vi "Enable Disable Controls.vi"(0 "Control Group 1":refnum<vi>[](array[refnum]), 5 "Control Group 2":refnum<vi>[](array[refnum]), 7 "Control Group 3":refnum<vi>[](array[refnum]), 11 "Error In":errorcluster, 12 "Visible / Hidden Control Group 3":bool, 13 "Control Group 2 Mode":T1(ring), 14 "Control Group 1 Mode":T1(ring)) -> (15 "Error Out":errorcluster)   [LabVIEW 2017, in "Waveform-Processing-Custom-Device System Explorer.lvlib"]
doc: "This will receive the reference array from the controls / indicators\nThe first 2 groups will disable/enable/gray/ the control\nThe last group will hide/show the control"
uses:
  Waveform-Processing-Custom-Device System Explorer.lvlib
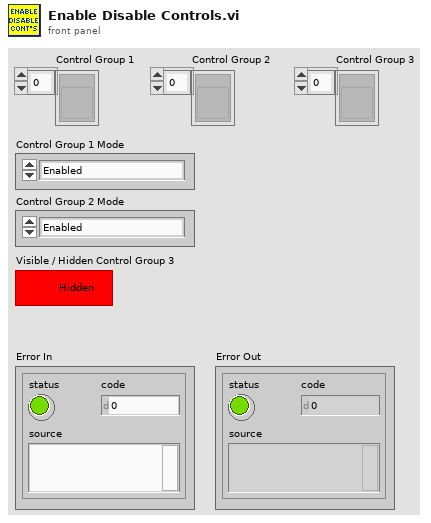
[diagram p1: front panel]
types:
  T1 = enum8{"Enabled", "Disabled", "Disabled and Grayed Out"}
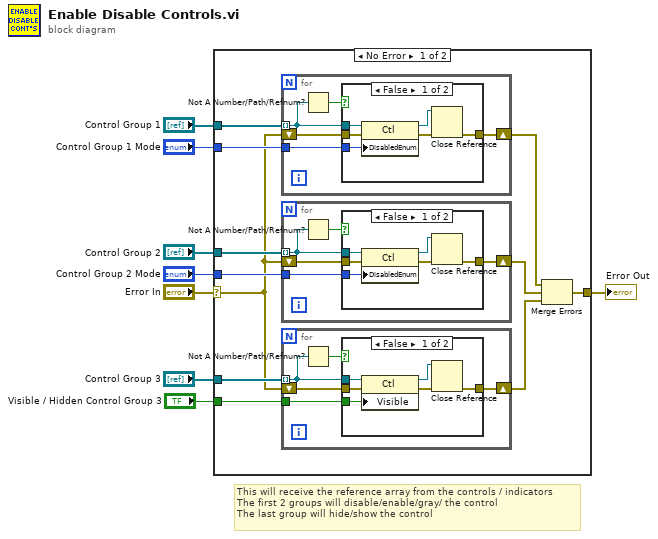
[diagram p0: block diagram]
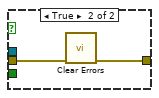
[diagram p2: hidden frame]
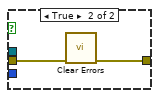
[diagram p3: hidden frame]
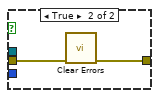
[diagram p4: hidden frame]
diagram:
  # "This will receive the reference array from the controls / indicators\nThe first 2 groups will disable/enable/gray/ the control\nThe last group will hide/show the control"
  n1 = case shown="No Error" "Error In" {
    selector: "Error In" -> [w14 w59]
    tunnel: "Control Group 1" -> [w19 _]
    tunnel: "Control Group 1 Mode" -> [w18 _]
    tunnel: "Control Group 2" -> [w17 _]
    tunnel: "Control Group 3" -> [w16 _]
    tunnel: "Control Group 2 Mode" -> [w15 _]
    tunnel: [w13 w59] -> w2
    tunnel: "Visible / Hidden Control Group 3" -> [w9 _]
    frame No Error {
      n2 = for {
        tunnel: w19 -> [w48] mode=indexing
        tunnel: w18 -> [w50]
        shift-right: [w46] -> w10
        shift-left: w14 -> [w49]
        n3 = Not A Number/Path/Refnum?(number/path/refnum=w48) -> (NaN/Path/Refnum?=w47:bool)
        n4 = case shown="False" w47 {
          tunnel: w50 -> [w54 _]
          tunnel: w49 -> [w53 w58]
          tunnel: w48 -> [w52 _]
          tunnel: [w51 w57] -> w46
          frame False {
            n5 = property class="Ctl"(reference=w52, error in=w53, "DisabledEnum"=w54) -> (reference out=w55:refnum<vi>, error out=w56:errorcluster)
            n6 = Close Reference(reference=w55, error in (no error)=w56) -> (error out=w51:errorcluster)
          }
          frame True {
            n7 = call <vilib>:"Clear Errors.vi"("error in (no error)"=w58) -> ("error out"=w57:errorcluster)  [unwired: 5 in, 1 out]
          }
        }
      }
      n8 = for {
        tunnel: w17 -> [w35] mode=indexing
        tunnel: w15 -> [w37]
        shift-right: [w33] -> w11
        shift-left: w14 -> [w36]
        n9 = Not A Number/Path/Refnum?(number/path/refnum=w35) -> (NaN/Path/Refnum?=w34:bool)
        n10 = case shown="False" w34 {
          tunnel: w37 -> [w41 _]
          tunnel: w36 -> [w40 w45]
          tunnel: w35 -> [w39 _]
          tunnel: [w38 w44] -> w33
          frame False {
            n11 = property class="Ctl"(reference=w39, error in=w40, "DisabledEnum"=w41) -> (reference out=w42:refnum<vi>, error out=w43:errorcluster)
            n12 = Close Reference(reference=w42, error in (no error)=w43) -> (error out=w38:errorcluster)
          }
          frame True {
            n13 = call <vilib>:"Clear Errors.vi"("error in (no error)"=w45) -> ("error out"=w44:errorcluster)  [unwired: 5 in, 1 out]
          }
        }
      }
      n14 = for {
        tunnel: w16 -> [w23] mode=indexing
        shift-right: [w21] -> w12
        shift-left: w14 -> [w24]
        tunnel: w9 -> [w20]
        n15 = Not A Number/Path/Refnum?(number/path/refnum=w23) -> (NaN/Path/Refnum?=w22:bool)
        n16 = case shown="False" w22 {
          tunnel: w24 -> [w28 w32]
          tunnel: w23 -> [w27 _]
          tunnel: [w26 w31] -> w21
          tunnel: w20 -> [w25 _]
          frame False {
            n17 = property class="Ctl"(reference=w27, error in=w28, "Visible"=w25) -> (reference out=w29:refnum<vi>, error out=w30:errorcluster)
            n18 = Close Reference(reference=w29, error in (no error)=w30) -> (error out=w26:errorcluster)
          }
          frame True {
            n19 = call <vilib>:"Clear Errors.vi"("error in (no error)"=w32) -> ("error out"=w31:errorcluster)  [unwired: 5 in, 1 out]
          }
        }
      }
      n20 = Merge Errors(w10, w11, w12) -> (w13:errorcluster)
    }
    frame Error {
    }
  }
  "Error Out" <- w2
